vi "add to subscribers list.vi"(8 "error in (no error)":errorcluster, 10 "Subscriber Data":T1, 11 "RSeries_CAM in":refnum<class "RSeries_CAM.lvclass">) -> (0 "error out":errorcluster, 3 "RSeries_CAM out":refnum<class "RSeries_CAM.lvclass">)   [LabVIEW 2024, in "RSeries_CAM.lvlib" / "RSeries_CAM.lvclass"]
uses:
  RSeries_CAM.lvclass
  ARCH/Message Queue/Message Cluster.ctl
  RSeries_CAM.lvclass/RSeries_CAM.ctl
  ARCH/Message Queue/Message Queue.lvlib
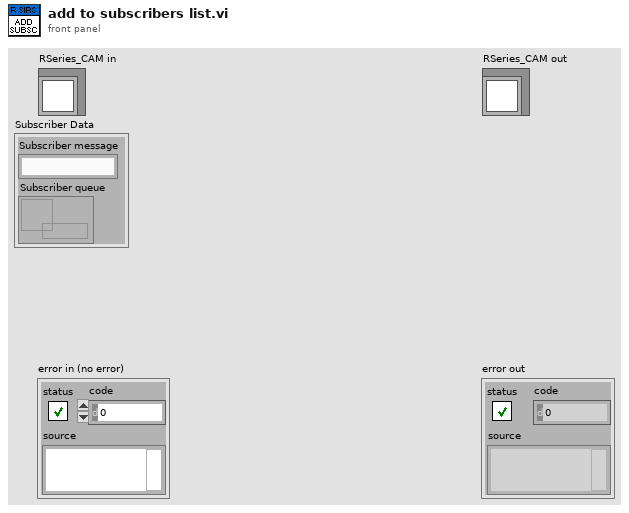
[diagram p1: front panel]
types:
  T1 = cluster{"Subscriber message":string, "Subscriber queue":refnum<queue>}
  T2 = cluster{"Subscriber message":string, "Subscriber queue":refnum<queue>}[]
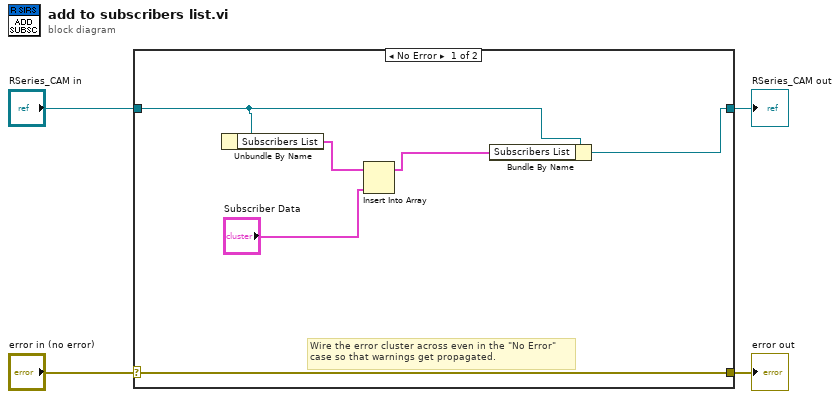
[diagram p0: block diagram]
diagram:
  n1 = case shown="No Error" "error in (no error)" {
    selector: "error in (no error)" -> [w10 w12]
    tunnel: [w10 w12] -> w3
    tunnel: [w5 w11] -> w1
    tunnel: "RSeries_CAM in" -> [w6 w11]
    frame No Error {
      # "Wire the error cluster across even in the \"No Error\"\ncase so that warnings get propagated."
      n2 = Unbundle By Name(w6) -> ("Subscribers List"=w9:T2)
      n3 = Insert Into Array(array=w9, new element="Subscriber Data") -> (w7:T2)  [unwired: 1 in]
      n4 = Bundle By Name(cluster=w6, "Subscribers List"=w7) -> (w5:refnum<class "RSeries_CAM.lvclass">)
    }
    frame Error {
    }
  }
  "error out" <- w3
  "RSeries_CAM out" <- w1
